vi "OpenFile.vi"(8 "error in (no error)":errorcluster, 11 "Measurement Directory":path) -> (0 "error out":errorcluster, 3 "File ref out":refnum<k34>)   [LabVIEW 2019]
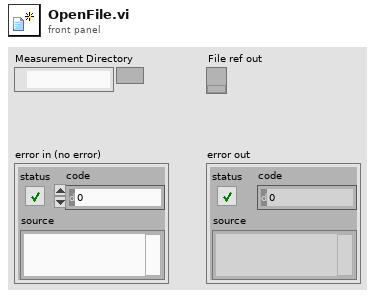
[diagram p1: front panel]
types:
  T1 = enum16{"open", "open or create", "create or replace", "create", "open (read-only)"}
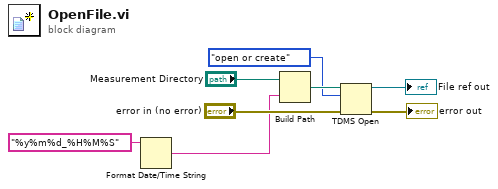
[diagram p0: block diagram]
diagram:
  n1 = Format Date/Time String(time format string (%c)="%y%m%d_%H%M%S") -> (date/time string=w4:string)  [unwired: 2 in]
  n2 = Build Path(base path="Measurement Directory", name or relative path=w4) -> (appended path=w3:path)
  n3 = TDMS Open(8:"error in (no error)", 10:T1."open or create" ("operation (0:open)"), 11:w3) -> (0:→"error out":errorcluster, 3:→"File ref out":refnum<k34>)  [unwired: 4 in]
